vi "Build Channel Cluster Array.vi"(0 "Cycler Cluster.lvclass in":refnum<class "Cycler Cluster.lvclass">, 1 "Channels Amount":u8) -> (7 "Channels out":cluster{"Channels":T1[]})   [LabVIEW 2023, in "Cycler Cluster.lvclass"]
uses:
  Cycler Cluster.lvclass
  Utilities/Channel.ctl
  Cycler Cluster.lvclass/Cycler Cluster.ctl
  Utilities/Utilities.lvlib
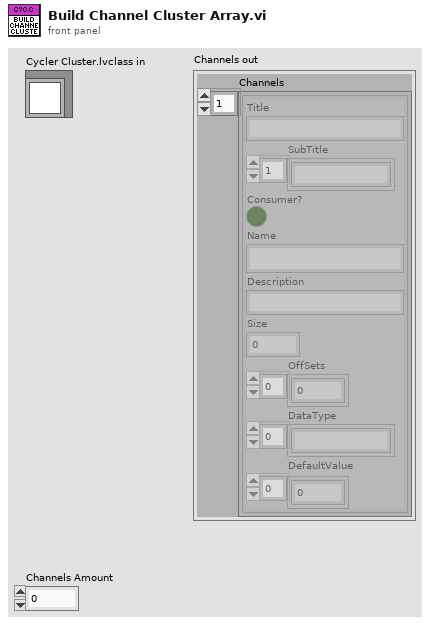
[diagram p1: front panel]
types:
  T1 = typedef "Utilities.lvlib/Channel.ctl" = cluster{"Title":string, "SubTitle":string[], "Consumer?":bool, "Name":string, "Description":string, "Size":i32, "OffSets":i32[], "DataType":string[], "DefaultValue":dbl[]}
  T2 = typedef "Cycler Cluster.lvclass/Consumer Control.ctl" = cluster{"OnOff.ACT":bool, "ErrorAcknowledge.ACT":bool, "IsoMeasurement.ACT":bool, "ParallelMode.ACT":bool}
  T3 = typedef "Cycler Cluster.lvclass/Producer Control.ctl" = cluster{"OnOff.STS":i32, "Error.STS":i32, "Watchdog.STS":i32, "IsoMeasurement.STS":i32, "ParallelMode.STS":i32}
  T4 = typedef "Cycler Cluster.lvclass/Consumer Ch.ctl" = cluster{"ErrorAcknowledge.ACT":bool, "OutputEnable.ACT":bool, "ControlMode.CTL":u16, "Voltage.SP":dbl, "VoltageMIN.SP":dbl, "VoltageMAX.SP":dbl, "VoltageGrad.SP":dbl, "Current.SP":dbl, "CurrentMIN.SP":dbl, "CurrentMAX.SP":dbl, "CurrentGrad.SP":dbl, "Power.SP":dbl, "PowerMIN.SP":dbl, "PowerMAX.SP":dbl, "PowerGrad.SP":dbl, "ParameterSet.CTL":i32}
  T5 = typedef "Cycler Cluster.lvclass/Producer Ch.ctl" = cluster{"Error.STS":i32, "OutputEnable.STS":i32, "ControlMode.STS":u16, "Voltage.AV":dbl, "Current.AV":dbl, "Power.AV":dbl, "VoltageNominal.AV":dbl, "CurrentNominal.AV":dbl, "PowerNominal.AV":dbl, "ParameterSet.STS":i32}
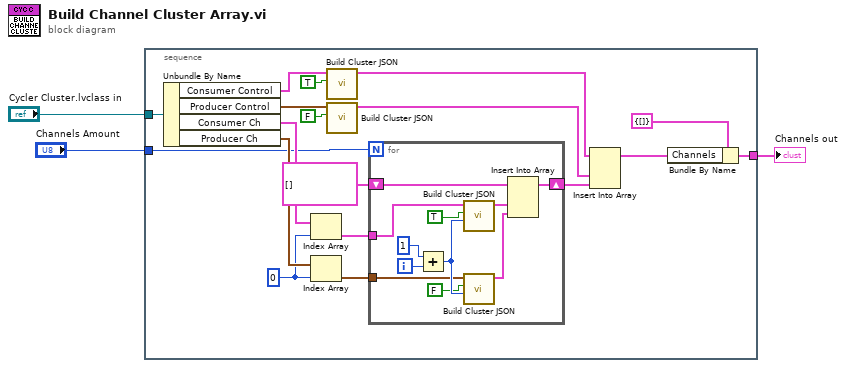
[diagram p0: block diagram]
diagram:
  n1 = stacked-sequence {
    tunnel: "Cycler Cluster.lvclass in" -> [w4]
    tunnel: "Channels Amount" -> [w16]
    tunnel: [w11] -> w1
    frame #0 {
      w19 = 0 ("index")
      n2 = Unbundle By Name(w4) -> ("Consumer Control"=w14:T2, "Producer Control"=w15:T3, "Consumer Ch"=w17:T4[], "Producer Ch"=w20:T5[])
      n3 = Index Array(array=w17, index=w19) -> (element=w18:T4)
      n4 = Index Array(array=w20, index=w19) -> (element=w21:T5)
      n5 = call "Build Cluster JSON.vi"("Consumer?"=TRUE, "Cluster"=w14) -> ("Array"=w7:T1[])  [unwired: 9 in]
      n6 = call "Build Cluster JSON.vi"("Consumer?"=FALSE, "Cluster"=w15) -> ("Array"=w8:T1[])  [unwired: 9 in]
      n7 = for {
        N: w16 -> [_]
        shift-right: [w28] -> w10
        shift-left: T1[] [] -> [w29]
        tunnel: w18 -> [w24]
        tunnel: w21 -> [w22]
        i -> [w27]
        n8 = Add(x=1, y=w27) -> (x+y=w25:i32)
        n9 = call "Build Cluster JSON.vi"("Channels Amount"=w25, "Consumer?"=TRUE, "Cluster"=w24) -> ("Array"=w31:T1[])  [unwired: 8 in]
        n10 = call "Build Cluster JSON.vi"("Channels Amount"=w25, "Consumer?"=FALSE, "Cluster"=w22) -> ("Array"=w30:T1[])  [unwired: 8 in]
        n11 = Insert Into Array(array=w29, new element #1=w31, new element #2=w30) -> (w28:T1[])  [unwired: 1 in]
      }
      n12 = Insert Into Array(array=w7, new element #1=w8, new element #2=w10) -> (w12:T1[])  [unwired: 1 in]
      n13 = Bundle By Name(cluster=cluster{"Channels":T1[]} {"Channels"=[]} ("Channels in"), "Channels"=w12) -> (w11:cluster{"Channels":T1[]})
    }
  }
  "Channels out" <- w1
